vi "shift wheel.vi"(6 "seq results name in":path, 9 "cycle results name in":path, 10 "Group run list write":string[][](array[string]), 11 "read write":string(combo)="read") -> (1 "cycle results name out":path, 2 "Group run list":string[][](array[string]), 4 "seq results name out":path)   [LabVIEW 2016]
doc: "This shift register is used to make changes to the wheel run order"
uses:
  <vilib>/Utility/file.llb/Read Delimited Spreadsheet (string).vi
  <vilib>/Utility/file.llb/Write Delimited Spreadsheet (string).vi
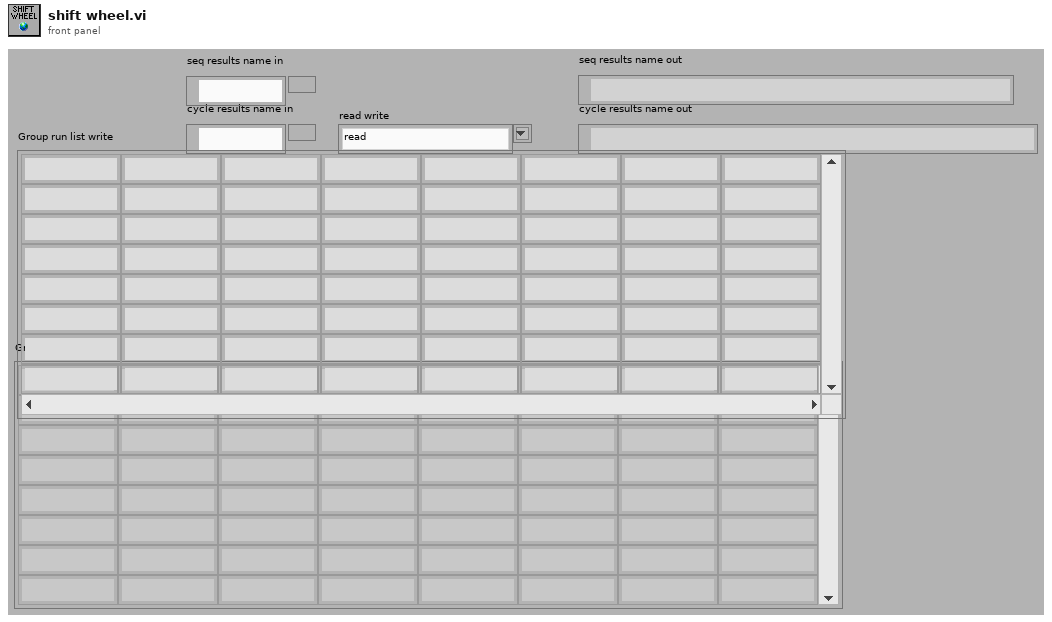
[diagram p1: front panel]
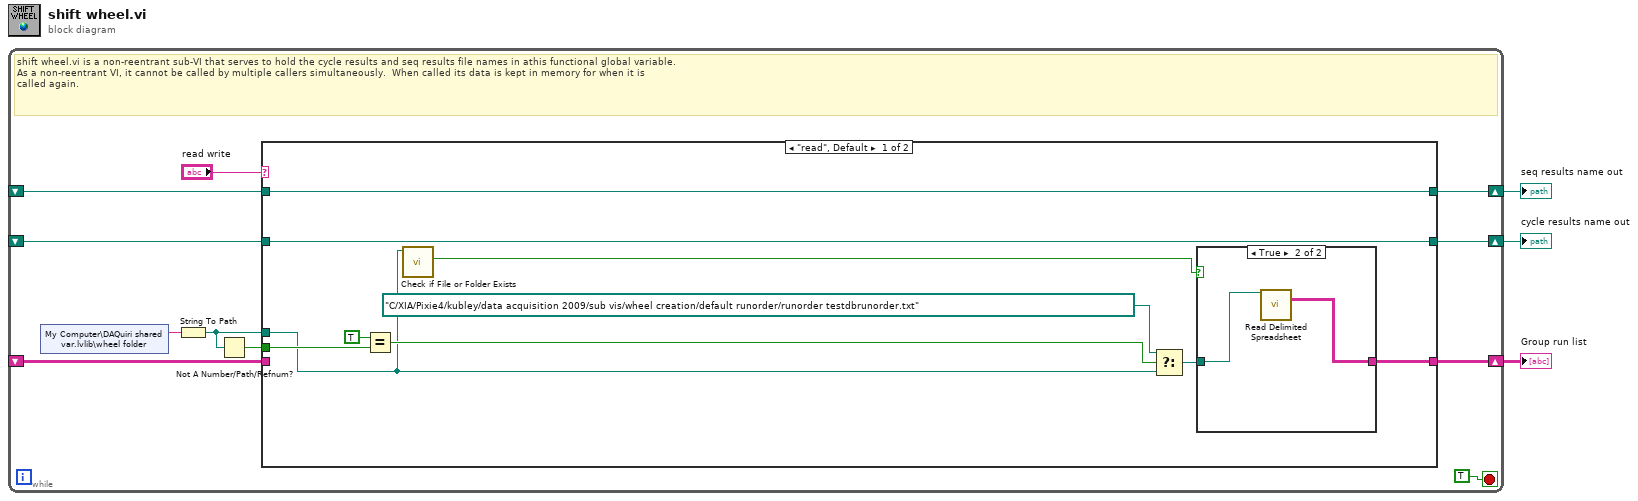
[diagram p0: block diagram]
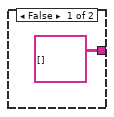
[diagram p2: hidden frame]
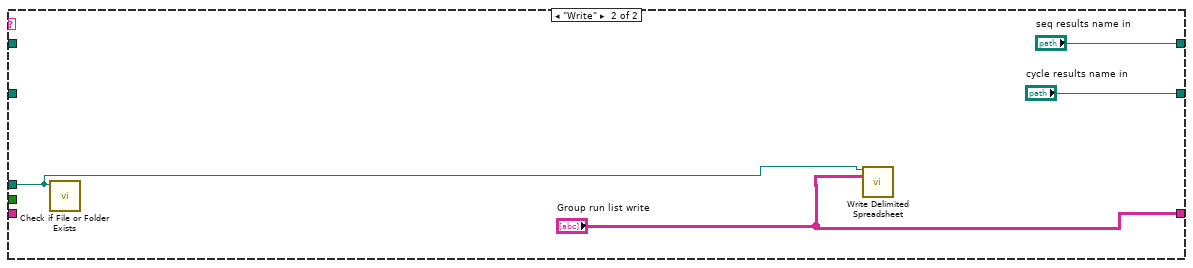
[diagram p3: hidden frame]
diagram:
  n1 = while {
    shift-right: [w13] -> w3
    shift-left: _ -> [w12]
    shift-right: [w10] -> w2
    shift-left: _ -> [w9]
    shift-right: [w8] -> w1
    shift-left: _ -> [w7]
    stop <- TRUE stop-if-true
    # "shift wheel.vi is a non-reentrant sub-VI that serves to hold the cycle results and seq results file names in athis functional global variable.\nAs a non-reentrant VI, it cannot be called by multiple callers simultaneously.  When called its data is kept in memory for when it is \ncalled again."
    n2 = shared-variable "My Computer\\DAQuiri shared var.lvlib\\wheel folder"() -> (w6:string)  [unwired: 1 in, 1 out]
    n3 = String To Path(string=w6) -> (path=w5:path)
    n4 = Not A Number/Path/Refnum?(number/path/refnum=w5) -> (NaN/Path/Refnum?=w4:bool)
    n5 = case shown="\"read\", Default" "read write" {
      tunnel: [w22 "Group run list write"] -> w13
      tunnel: w12 -> [_ _]
      tunnel: [w24 "cycle results name in"] -> w10
      tunnel: w9 -> [w24 _]
      tunnel: [w23 "seq results name in"] -> w8
      tunnel: w7 -> [w23 _]
      tunnel: w5 -> [w16 w28]
      tunnel: w4 -> [w21 _]
      frame "read", Default {
        n6 = Equal?(x=TRUE, y=w21) -> (x = y?=w19:bool)
        n7 = call <vilib>:"Check if File or Folder Exists.vi"("path"=w16) -> ("file or folder exists?"=w15:bool)  [unwired: 8 in, 2 out]
        n8 = Select(t=path "C:/XIA/Pixie4/kubley/data acquisition 2009/sub vis/wheel creation/default runorder/runorder testdbrunorder.txt", s=w19, f=w16) -> (s? t:f=w17:path)
        n9 = case shown="True" w15 {
          tunnel: [string[][] [] ("all rows") w27] -> w22
          tunnel: w17 -> [_ w26]
          frame False {
          }
          frame True {
            n10 = call-poly <vilib>:"Read Delimited Spreadsheet.vi"("file path (dialog if empty)"=w26) -> ("all rows"=w27:string[][])  [unwired: 9 in, 5 out]
          }
        }
      }
      frame "Write" {
        n11 = call <vilib>:"Check if File or Folder Exists.vi"("path"=w28) -> ()  [unwired: 8 in, 3 out]
        n12 = call-poly <vilib>:"Write Delimited Spreadsheet.vi"("file path (dialog if empty)"=w28, "2D data"="Group run list write") -> ()  [unwired: 12 in, 2 out]
      }
    }
  }
  "Group run list" <- w3
  "cycle results name out" <- w2
  "seq results name out" <- w1
